vi "Caculator.vi"(7 "DATA":i16[](array[numeric]), 8 "error in (no error)":errorcluster, 11 "Caculator in":refnum<class "Caculator.lvclass">) -> (0 "error out":errorcluster, 2 "Waveform Graph":waveform(dbl)[](graph), 3 "Caculator out":refnum<class "Caculator.lvclass">)   [LabVIEW 2017, in "Caculator.lvclass"]
uses:
  Caculator.lvclass
  Caculator.lvclass/Caculator.ctl
  <vilib>/measure/madcrms.llb/Basic Averaged DC-RMS for 1 Chan.vi
  <vilib>/measure/NI_MAPro.lvlib
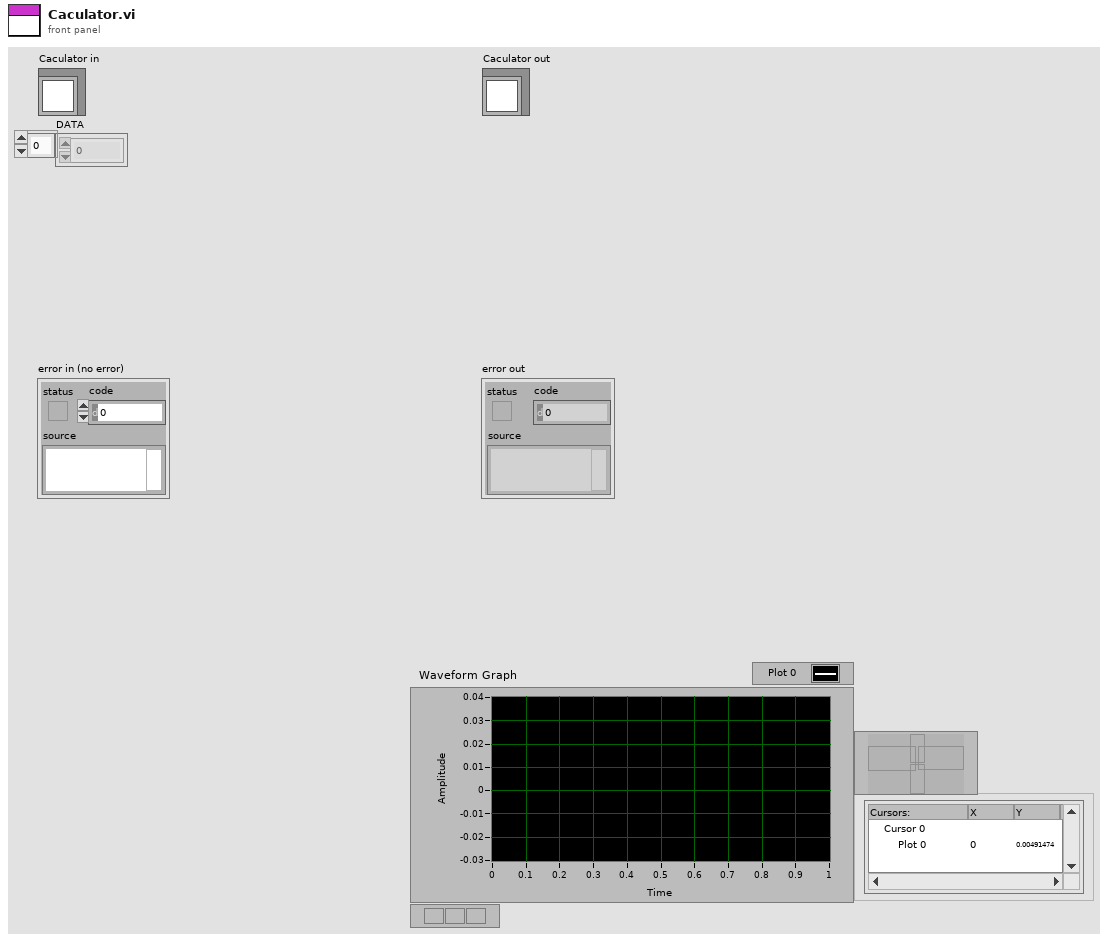
[diagram p1: front panel]
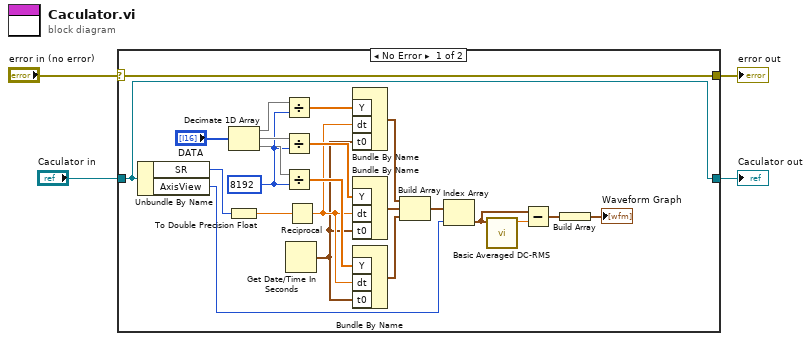
[diagram p0: block diagram]
diagram:
  n1 = case shown="No Error" "error in (no error)" {
    selector: "error in (no error)" -> [w27 w29]
    tunnel: [w27 w29] -> w3
    tunnel: [w11 w28] -> w1
    tunnel: "Caculator in" -> [w11 w28]
    frame No Error {
      w20 = 8192 ("length")
      n2 = Unbundle By Name(w11) -> ("SR"=w26:u16, "AxisView"=w9:enum16{"X", "Y", "Z"})
      n3 = Decimate 1D Array("DATA") -> (w24:i16[], w22:i16[], w21:i16[])
      n4 = To Double Precision Float(number=w26) -> (double precision float=w25:dbl)
      n5 = Divide(x=w24, y=w20) -> (x/y=w19:dbl[])
      n6 = Divide(x=w22, y=w20) -> (x/y=w18:dbl[])
      n7 = Divide(x=w21, y=w20) -> (x/y=w17:dbl[])
      n8 = Get Date/Time In Seconds() -> (seconds since 1Jan1904=w12:timestamp)
      n9 = Reciprocal(x=w25) -> (1/x=w16:dbl)
      n10 = Bundle By Name("Y"=w19, "dt"=w16, "t0"=w12) -> (w15:waveform(dbl))  [unwired: 1 in]
      n11 = Bundle By Name("Y"=w18, "dt"=w16, "t0"=w12) -> (w14:waveform(dbl))  [unwired: 1 in]
      n12 = Bundle By Name("Y"=w17, "dt"=w16, "t0"=w12) -> (w13:waveform(dbl))  [unwired: 1 in]
      n13 = Build Array(w15, w14, w13) -> (w5:waveform(dbl)[])
      n14 = Index Array(array=w5, index=w9) -> (element=w7:waveform(dbl))
      n15 = call-poly <vilib>:"Basic Averaged DC-RMS.vi"("signal in"=w7) -> ("DC value"=w8:dbl)  [unwired: 7 in, 3 out]
      n16 = Subtract(x=w7, y=w8) -> (x-y=w6:waveform(dbl))
      n17 = Build Array(w6) -> (→"Waveform Graph":waveform(dbl)[])
    }
    frame Error {
    }
  }
  "error out" <- w3
  "Caculator out" <- w1
